vi "基础18.vi"() -> ()   [LabVIEW 2014]
uses:
  <vilib>/express/express analysis/Spectral/Block/exnSpectralBlock spectral measurements power poly.vi
  <vilib>/express/express analysis/Spectral/Block/exnSpectralBlock spectral measurements power DDT.vi
  <vilib>/express/express analysis/Spectral/XNode/ExpressSpectralMeasurementsBlockNode.xnode
panel:
  out "波形图表 2":dynamicdata(graph)
  in  "停止":bool
  out "波形图表":dynamicdata(graph)
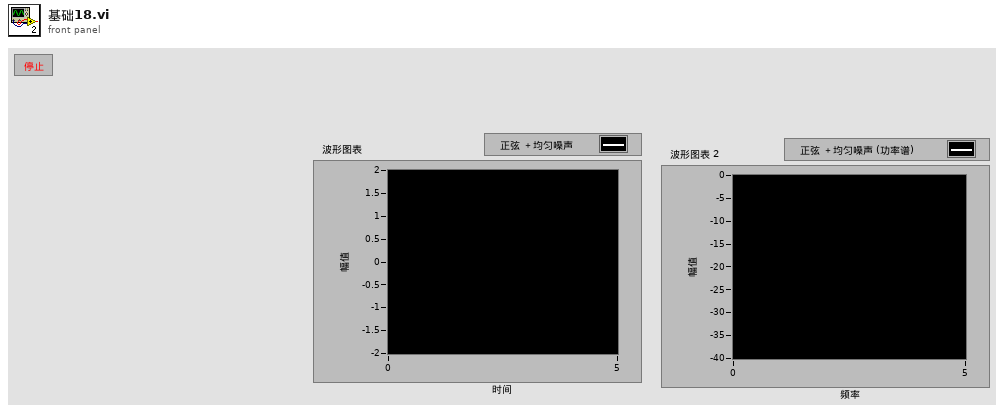
[diagram p1: front panel]
types:
  T1 = cluster{"averaging mode":u16, "weighting mode":u16, "number of averages":u32}
  T2 = cluster{"dB On (F)":bool, "unwrap phase (F)":bool, "convert to degree (F)":bool}
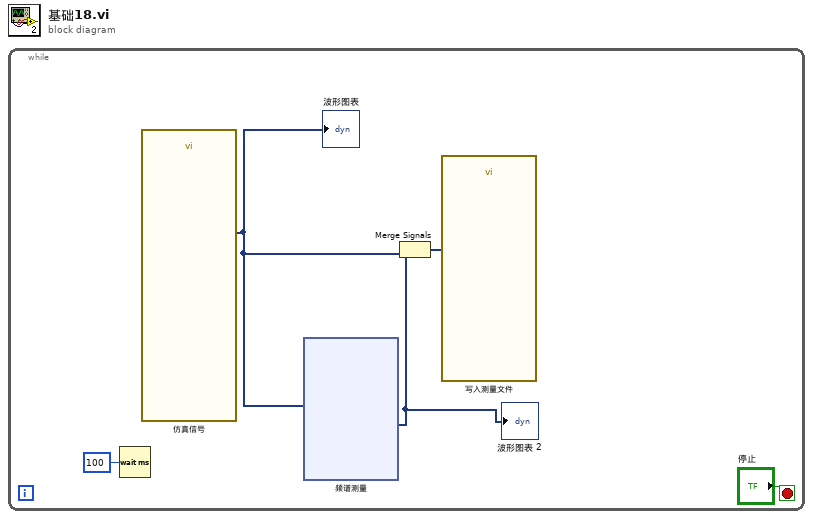
[diagram p0: block diagram]
diagram:
  n1 = while {
    stop <- "停止" stop-if-true
    n2 = Wait (ms)(milliseconds to wait=u32 100 ("等待时间（毫秒）")) -> ()  [unwired: 1 out]
    n3 = call "仿真信号"() -> ("正弦与均匀噪声"=w3:dynamicdata)  [unwired: 14 in, 1 out]
    "波形图表" <- w3
    n4 = xnode "频谱测量"("信号"=w3) -> ("功率谱"=w2:dynamicdata)  [unwired: 1 in, 1 out]
    "波形图表 2" <- w2
    n5 = Merge Signals(w2, w3) -> (w4:dynamicdata)
    n6 = call "写入测量文件"("Signals"=w4) -> ()  [unwired: 16 in, 3 out]
  }
